vi "SignalGenerator.vi"(10 "Frequency":i32, 11 "Amplitude":i32=2) -> (3 "Input signal":dbl)   [LabVIEW 2014]
panel:
  out "error out 2":errorcluster caption="error out"
  in  "error in (no error)":errorcluster
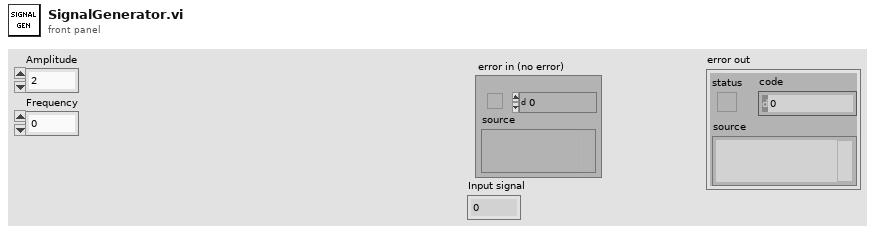
[diagram p1: front panel]
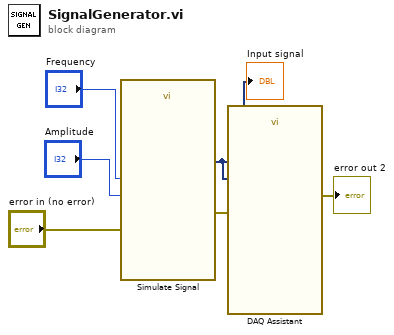
[diagram p0: block diagram]
diagram:
  n1 = call "Simulate Signal"("Frequency"="Frequency", "Amplitude"="Amplitude", "error in (no error)"="error in (no error)") -> ("Sine"=w1:dynamicdata, "error out"=w3:errorcluster)  [unwired: 11 in]
  "Input signal" <- w1
  n2 = call "DAQ Assistant"("data"=w1, "error in"=w3) -> ("error out"=→"error out 2":errorcluster)  [unwired: 15 in, 2 out]
